vi "NML Data Acq Globals.vi"() -> ()   [LabVIEW 2024]
panel:
  in  "Instrument Name Adjustments":cluster{"Test":string, "Replacement":string}[](array[cluster])=[{"Test"="HEWLETT-PACKARD", "Replacement"="HP"}, {"Test"="KEITHLEY INSTRUMENTS INC.", "Replacement"="Keithley"}, {"Test"="ANDEEN-HAGERLING", "Replacement"="AH"}, {"Test"="Stanford_Research_Systems", "Replacement"="SRS"}, {"Test"="StanfordResearchSystems", "Replacement"="SRS"}, {"Test"="KEITHLEY INSTRUMENTS", "Replacement"="Keithley"}]
  in  "Strings To Remove from IDN":string[](array[string])=["MANUFACTURER", "MODEL/OPTIONS", "SERIAL NUMBER", "ACTIVE FIRMWARE", "----", "C---"]
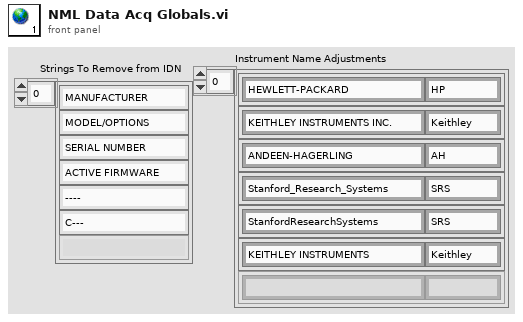
[diagram p1: front panel]
diagram:
